vi "ROS_Topic_Write.vi"(3 "error in (no error)":errorcluster, 4 "Msg in":string, 5 "ROS in":T1={"topic port"=0, "Node"="", "topic"="", "type"="", "node port"=0, "error "={"status"=FALSE, "code"=0, "source"=""}, "Direction"=enum."Node", "Update (ms)"=1, "FIFO size"=1}) -> (0 "error out":errorcluster, 2 "ROS out":T1={"topic port"=0, "Node"="", "topic"="", "type"="", "node port"=0, "error "={"status"=FALSE, "code"=0, "source"=""}, "Direction"=enum."Node", "Update (ms)"=1, "FIFO size"=1})   [LabVIEW 2012]
doc: "Prepends the length to Msg in before sending out the data on the specified topic. Use only for publishers and service clients. Messages need to be formatted using Message Building functionality. \n\nSetting Continuous to True will instruct the server to publish the message it received as quickly as possible, updating the message when a new ROS_Topic_Write is called."
uses:
  SubVIs/_ROSControl.ctl
  SubVIs/_ROSDirection.ctl
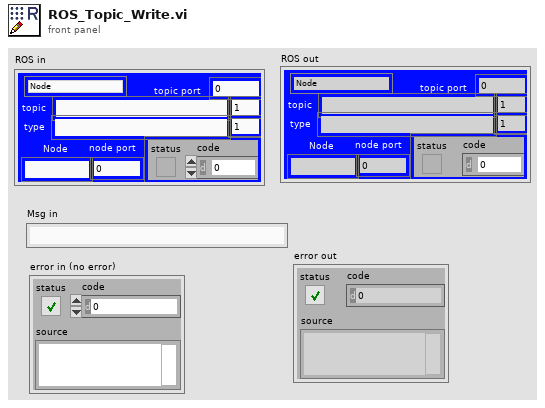
[diagram p1: front panel]
types:
  T1 = typedef "_ROSControl.ctl" = cluster{"topic port":u16, "Node":string, "topic":string, "type":string, "node port":u16, "error ":errorcluster, "Direction":T2, "Update (ms)":u16, "FIFO size":u16}
  T2 = typedef "_ROSDirection.ctl" = enum16{"Node", "Publisher", "Subscriber", "ServiceClient", "ServiceProvider"}
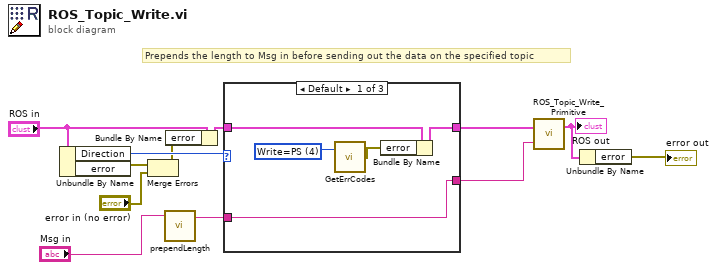
[diagram p0: block diagram]
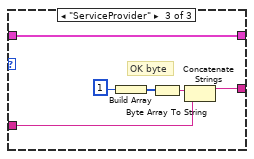
[diagram p3: hidden frame]
diagram:
  # "Prepends the length to Msg in before sending out the data on the specified topic"
  n1 = Unbundle By Name("ROS in") -> ("Direction"=w12:T2, "error"=w11:errorcluster)
  n2 = Merge Errors(w11, "error in (no error)") -> (w8:errorcluster)
  n3 = call "prependLength.vi"("msg in"="Msg in") -> ("msg out"=w1:string)  [unwired: 4 in]
  n4 = Bundle By Name(cluster="ROS in", "error"=w8) -> (w9:T1)
  n5 = case shown="Default" w12 {
    tunnel: [w17 w19 w25] -> w4
    tunnel: w9 -> [w16 w19 w25]
    tunnel: [w15 w18 w23] -> w3
    tunnel: w1 -> [w15 w18 w24]
    frame Default {
      w13 = u16 4 items=["TopicReadTimeout", "Read=SS", "GetQueueErr", "NoMaster", "Write=PS"] ("Error")
      n6 = call "GetErrCodes.vi"("Error"=w13) -> ("Error"=w14:errorcluster)  [unwired: 1 in]
      n7 = Bundle By Name(cluster=w16, "error"=w14) -> (w17:T1)
    }
    frame "Publisher", "ServiceClient" {
    }
    frame "ServiceProvider" {
      # "OK byte"
      n8 = Build Array(u8 1 ("Numeric")) -> (w20:u8[])
      n9 = Byte Array To String(unsigned byte array=w20) -> (string=w22:string)
      n10 = Concatenate Strings(w22, w24) -> (w23:string)
    }
  }
  n11 = call "ROS_Topic_Write_Primitive.vi"("Msg in"=w3, "ROS in"=w4) -> ("ROS out"=w5:T1)  [unwired: 1 in]
  "ROS out" <- w5
  n12 = Unbundle By Name(w5) -> ("error"=→"error out":errorcluster)
